vi "Manual Control (Global).vi"() -> ()   [LabVIEW 2018]
panel:
  in  "SOC":dbl=50.0
  in  "Manual PCC":bool=TRUE
  in  "Load P Setpoint":dbl[](array[numeric])=[50.0, 50.0, 50.0]
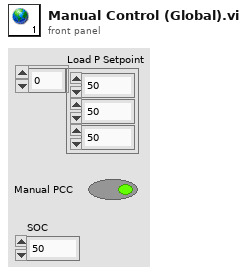
[diagram p1: front panel]
diagram:
